vi "Clear.vi"(8 "error in (no error)":errorcluster, 9 "offset (0)":u64 format="%d bytes", 10 "length (-1: rest)":i64=-1 format="%d bytes", 11 "Pointer in":refnum<class "Pointer.lvclass">) -> (0 "error out":errorcluster, 3 "Pointer out":refnum<class "Pointer.lvclass">)   [LabVIEW 2020, in "Memory Manager.lvlib" / "Pointer.lvclass"]
doc: "Sets the subset of bytes specified by <b>offset</b> and <b>length</b> for <b>Pointer</b> to zero."
uses:
  Pointer.lvclass
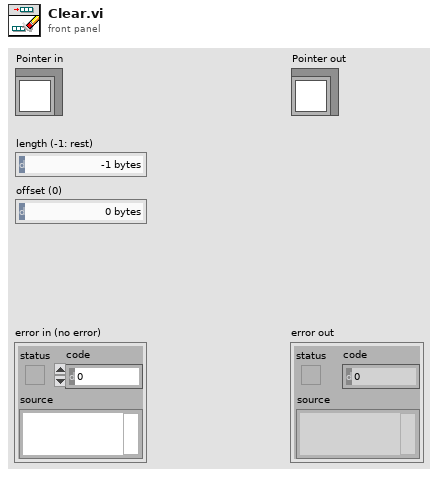
[diagram p1: front panel]
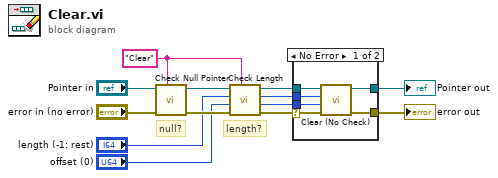
[diagram p0: block diagram]
diagram:
  w5 = "Clear" ("source vi name")
  # "length?"
  # "null?"
  n1 = call "Check Null Pointer.vi"("source vi name"=w5, "error in (no error)"="error in (no error)", "Pointer in"="Pointer in") -> ("error out"=w8:errorcluster, "Pointer out"=w9:refnum<class "Pointer.lvclass">)  [unwired: 7 in]
  n2 = call "Check Length.vi"("source vi name"=w5, "error in (no error)"=w8, "offset (0)"="offset (0)", "length (-1: rest)"="length (-1: rest)", "Pointer in"=w9) -> ("error out"=w6:errorcluster, "offset"=w3:u64, "size"=w4:u64, "Pointer out"=w7:refnum<class "Pointer.lvclass">)  [unwired: 3 in]
  n3 = case shown="No Error" w6 {
    selector: w6 -> [w14 w20]
    tunnel: w7 -> [w19 w21]
    tunnel: w4 -> [w18 _]
    tunnel: w3 -> [w17 _]
    tunnel: [w16 w21] -> w11
    tunnel: [w15 w20] -> w10
    frame No Error {
      n4 = call "Clear (No Check).vi"("error in (no error)"=w14, "offset (0)"=w17, "size"=w18, "Pointer in"=w19) -> ("error out"=w15:errorcluster, "Pointer out"=w16:refnum<class "Pointer.lvclass">)  [unwired: 6 in]
    }
    frame Error {
    }
  }
  "error out" <- w10
  "Pointer out" <- w11
